vi "Report_StringIsURL.vi"(8 "error in (no error)":errorcluster, 11 "String":string) -> (0 "error out":errorcluster, 3 "Is URL?":bool)   [LabVIEW 2017, in "NI_ReportGenerationCore.lvlib"]
doc: "Checks if the string begins with a recognized URL prefix."
uses:
  <vilib>/Utility/NIReport.llb/NI_ReportGenerationCore.lvlib
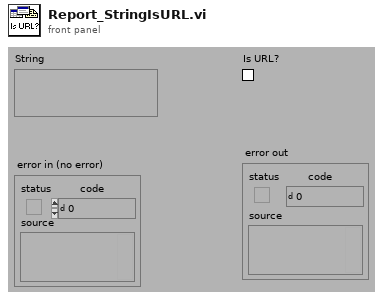
[diagram p1: front panel]
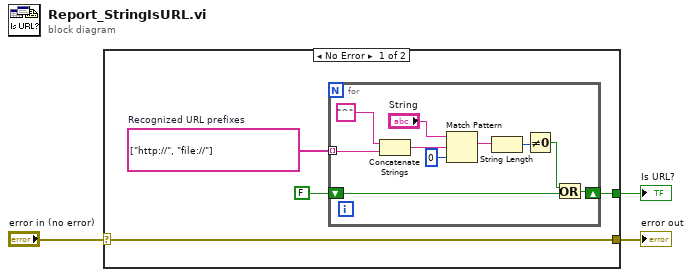
[diagram p0: block diagram]
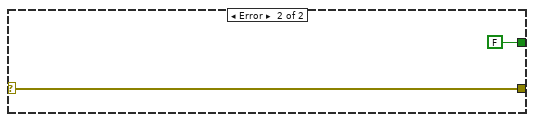
[diagram p2: hidden frame]
diagram:
  n1 = case shown="No Error" "error in (no error)" {
    selector: "error in (no error)" -> [w5 w19]
    tunnel: [w5 w19] -> w2
    tunnel: [w4 FALSE] -> w1
    frame No Error {
      w7 = string[] ["http://", "file://"]  # Recognized URL prefixes
      n2 = for {
        tunnel: w7 -> [w15] mode=indexing
        shift-right: [w9] -> w4
        shift-left: FALSE -> [w8]
        n3 = Concatenate Strings("^", w15) -> (w14:string)
        n4 = Match Pattern(string="String", regular expression=w14, offset (0)=0) -> (match substring=w12:string)  [unwired: 3 out]
        n5 = String Length(string=w12) -> (length=w11:i32)
        n6 = Not Equal To 0?(x=w11) -> (x != 0?=w10:bool)
        n7 = Or(x=w10, y=w8) -> (x .or. y?=w9:bool)
      }
    }
    frame Error {
    }
  }
  "error out" <- w2
  "Is URL?" <- w1
